vi "GetChainNumbersFromMask.vi"(1 "ChainMask":u8 format="0x%02x") -> (0 "Chains":u8[](array[numeric]))   [LabVIEW 2018, in "ArduinoSerialBling.lvlib"]
uses:
  ArduinoSerialBling.lvlib
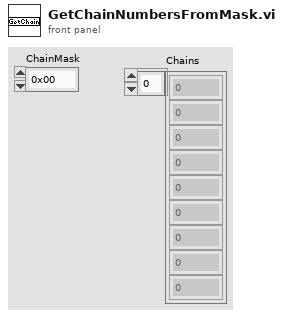
[diagram p1: front panel]
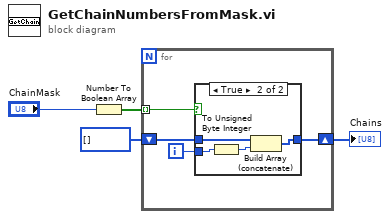
[diagram p0: block diagram]
diagram:
  n1 = Number To Boolean Array(number="ChainMask") -> (Boolean array=w3:bool[])
  n2 = for {
    tunnel: w3 -> [w7] mode=indexing
    shift-right: [w5] -> w1
    shift-left: u8[] [] -> [w8]
    i -> [w6]
    n3 = case shown="True" w7 {
      tunnel: w8 -> [w9 w13]
      tunnel: w6 -> [_ w12]
      tunnel: [w9 w11] -> w5
      frame False {
      }
      frame True {
        n4 = To Unsigned Byte Integer(number=w12) -> (unsigned 8bit integer=w10:u8)
        n5 = Build Array (concatenate)(w13, w10) -> (w11:u8[])
      }
    }
  }
  "Chains" <- w1
